vi "AG33XXX.initialize.vi"(0 "i ref in":refnum<vi>, 1 "queryID":bool, 2 "resetDevice":bool, 3 "ms timeout (10000)":i32=10000, 5 "error in (no error)":errorcluster) -> (14 "i ref out":refnum<vi>, 16 "deviceID":string, 17 "timed out":bool, 19 "error out":errorcluster)   [LabVIEW 2014, in "AG33XXX.lvlib"]
doc: "(Re)initializs the device."
uses:
  AG33XXX.lvlib
  CS_Core/CSApplicationBaseClasses/DeviceBase/DeviceBase.lvlib
  instr.lib/agilent_33xxx_series/Agilent 33XXX Series/Agilent 33XXX Series.lvlib
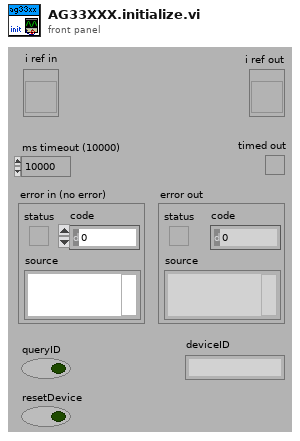
[diagram p1: front panel]
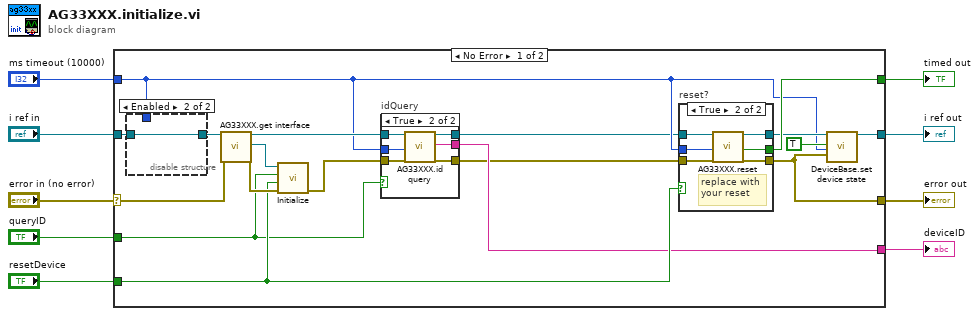
[diagram p0: block diagram]
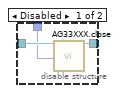
[diagram p2: hidden frame]
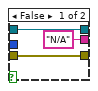
[diagram p3: hidden frame]
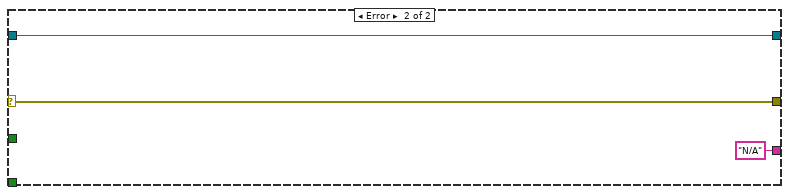
[diagram p5: hidden frame]
diagram:
  n1 = case shown="No Error" "error in (no error)" {
    selector: "error in (no error)" -> [w20 w50]
    tunnel: [w27 _] -> w9
    tunnel: [w24 w51] -> w8
    tunnel: "ms timeout (10000)" -> [w14 _]
    tunnel: "i ref in" -> [w26 w51]
    tunnel: "queryID" -> [w13 _]
    tunnel: [w22 w50] -> w3
    tunnel: "resetDevice" -> [w17 _]
    tunnel: [w12 "N/A"] -> w1
    frame No Error {
      n2 = disable-structure shown="Enabled" {
        disable-tunnel: w26 -> [w30 w31]
        disable-tunnel: [w29 w31] -> w21
        disable-tunnel: w14 -> [w28 _]
        frame Disabled {
          n3 = call "AG33XXX.close.vi"("i ref in"=w30, "ms timeout (10000)"=w28) -> ("i ref out"=w29:refnum<vi>)  [unwired: 15 in, 2 out]
        }
        frame Enabled {
        }
      }
      n4 = call "AG33XXX.get interface.vi"("i ref in"=w21, "error in (no error)"=w20) -> ("i ref out"=w16:refnum<vi>, "interface"=w19:refnum<visa-resource-name>, "error out"=w18:errorcluster)  [unwired: 15 in]
      n5 = call "Initialize.vi"("error in (no error)"=w18, "Reset? (T: Yes)"=w17, "ID Query? (T: Yes)"=w13, "VISA resource name"=w19) -> ("error out"=w15:errorcluster)  [unwired: 6 in, 1 out]
      n6 = case "idQuery" shown="True" w13 {
        tunnel: w16 -> [w34 w40]
        tunnel: w15 -> [w33 w39]
        tunnel: w14 -> [_ w38]
        tunnel: [w34 w37] -> w11
        tunnel: [w33 w36] -> w10
        tunnel: ["N/A" ("IDString") w35] -> w12
        frame False {
        }
        frame True {
          n7 = call "AG33XXX.id query.vi"("i ref in"=w40, "ms timeout (10000)"=w38, "error in (no error)"=w39) -> ("i ref out"=w37:refnum<vi>, "IDString"=w35:string, "error out"=w36:errorcluster)  [unwired: 13 in, 1 out]
        }
      }
      n8 = case "reset?" shown="True" w17 {
        tunnel: w11 -> [w42 w48]
        tunnel: w10 -> [w41 w47]
        tunnel: w14 -> [_ w46]
        tunnel: [_ w45] -> w27
        tunnel: [w41 w44] -> w22
        tunnel: [w42 w43] -> w25
        frame False {
        }
        frame True {
          # "replace with\nyour reset"
          n9 = call "AG33XXX.reset.vi"("i ref in"=w48, "ms timeout (10000)"=w46, "error in (no error)"=w47) -> ("i ref out"=w43:refnum<vi>, "timed out"=w45:bool, "error out"=w44:errorcluster)  [unwired: 14 in]
        }
      }
      n10 = call "DeviceBase.set device state.vi"("i ref in"=w25, "implicit"=TRUE, "ms timeout (10000)"=w14, "device error"=w22) -> ("i ref out"=w24:refnum<vi>)  [unwired: 13 in, 2 out]
    }
    frame Error {
    }
  }
  "error out" <- w3
  "i ref out" <- w8
  "timed out" <- w9
  "deviceID" <- w1
